vi "get_19052_AC_step_test_time.vi"(8 "error in (no error)":errorcluster, 10 "Step":u16=1 min=1 max=99 step=1, 11 "VISA resource in":refnum<visa-resource-name>) -> (0 "error out":errorcluster, 2 "AC total time":string, 3 "VISA resource out":refnum<visa-resource-name>)   [LabVIEW 2015]
doc: "This VI retrieves the test TIME of the selected step and mode."
uses:
  Type Definitions/get_19052_AC_step_time_states.ctl
  Type Definitions/ac_dc_ir_control.ctl
panel:
  # "Get 19052 AC test time"
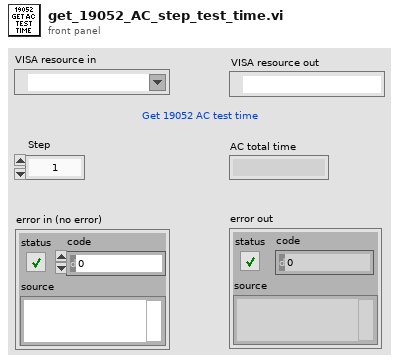
[diagram p1: front panel]
types:
  T1 = typedef "get_19052_AC_step_time_states.ctl" = enum16{"Initilize", "get RAMP time", "get TIME", "get FALL time", "calc TOTAL time", "Error", "Shutdown"}
  T2 = cluster{"ramp time":dbl, "time":dbl, "fall time":dbl, "total time":string}
  T3 = typedef "ac_dc_ir_control.ctl" = enum16{"AC", "DC", "IR"}
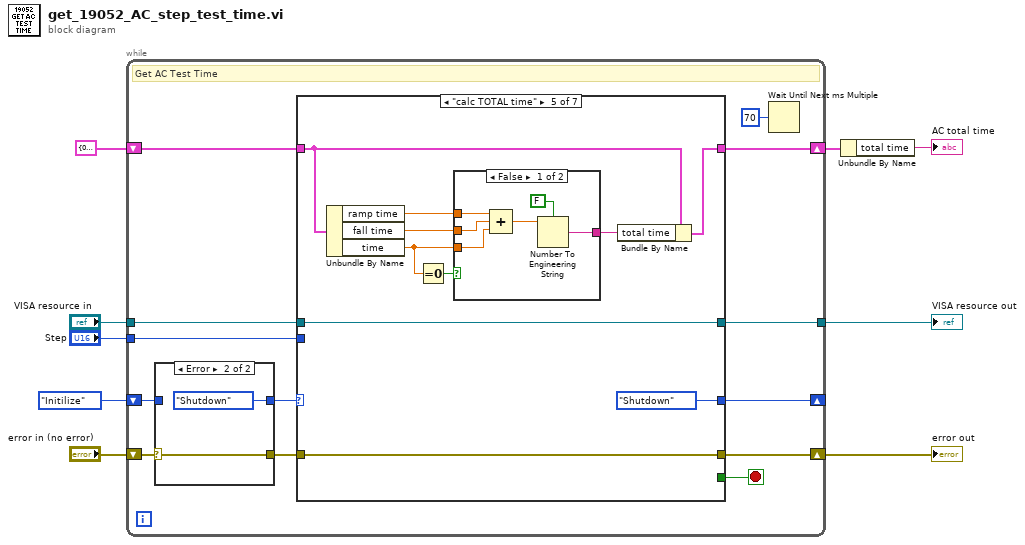
[diagram p0: block diagram]
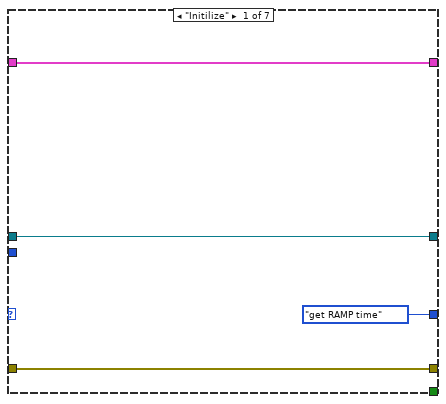
[diagram p3: hidden frame]
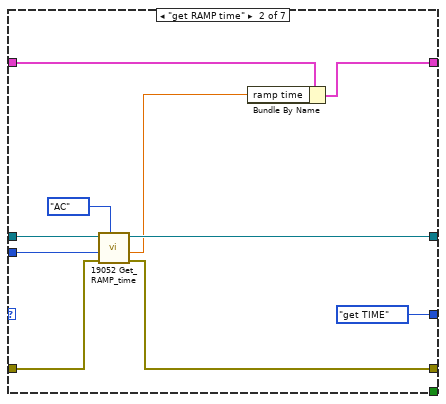
[diagram p4: hidden frame]
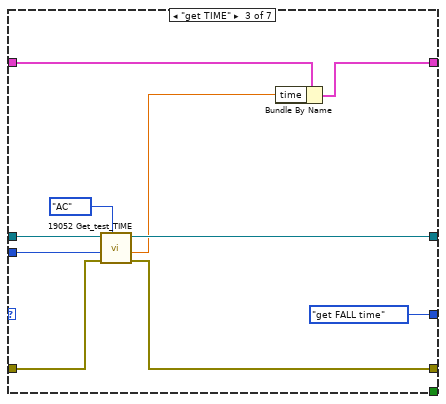
[diagram p5: hidden frame]
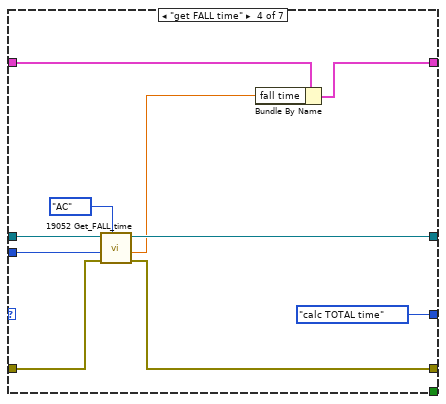
[diagram p6: hidden frame]
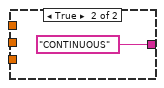
[diagram p7: hidden frame]
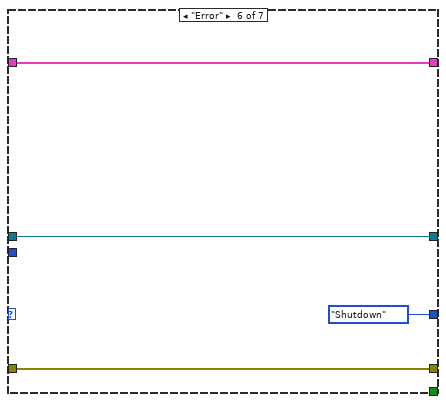
[diagram p8: hidden frame]
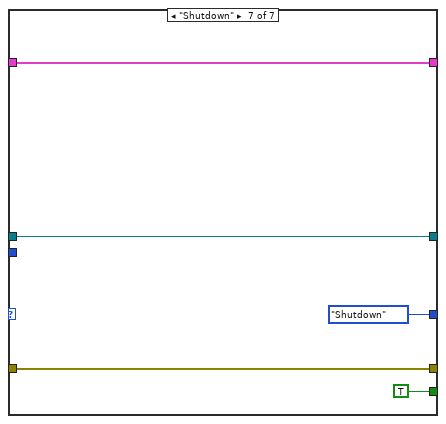
[diagram p9: hidden frame]
diagram:
  n1 = while {
    shift-right: [w22] -> _
    shift-left: get_19052_AC_step_time_states."Initilize" ("States") -> [w13]
    tunnel: "VISA resource in" -> [w21]
    tunnel: [w20] -> w6
    shift-right: [w19] -> w8
    shift-left: "error in (no error)" -> [w16]
    shift-right: [w17] -> w2
    shift-left: T2 {"ramp time"=0.0, "time"=0.0, "fall time"=0.0, "total time"=""} -> [w18]
    tunnel: "Step" -> [w12]
    stop <- w11 stop-if-true
    # "Get AC Test Time"
    n2 = case shown="Error" w16 {
      selector: w16 -> [w24 w26]
      tunnel: [w24 w26] -> w15
      tunnel: [w23 get_19052_AC_step_time_states."Shutdown" ("States")] -> w14
      tunnel: w13 -> [w23 _]
      frame No Error {
      }
      frame Error {
      }
    }
    n3 = case shown="\"calc TOTAL time\"" w14 {
      tunnel: [get_19052_AC_step_time_states."get RAMP time" ("States") get_19052_AC_step_time_states."get TIME" ("States") get_19052_AC_step_time_states."get FALL time" ("States") get_19052_AC_step_time_states."calc TOTAL time" ("States") get_19052_AC_step_time_states."Shutdown" ("States") get_19052_AC_step_time_states."Shutdown" ("States") get_19052_AC_step_time_states."Shutdown" ("States")] -> w22
      tunnel: w21 -> [w30 w39 w48 w58 w70 w81 w86]
      tunnel: [w30 w38 w46 w56 w70 w81 w86] -> w20
      tunnel: w15 -> [w29 w37 w47 w57 w69 w80 w85]
      tunnel: [w29 w36 w45 w55 w69 w80 w85] -> w19
      tunnel: w18 -> [w28 w40 w50 w60 w66 w79 w84]
      tunnel: [w28 w34 w49 w59 w67 w79 w84] -> w17
      tunnel: w12 -> [_ w35 w44 w54 _ _ _]
      tunnel: [_ _ _ _ _ _ TRUE] -> w11
      frame "Initilize" {
      }
      frame "get RAMP time" {
        n4 = call "19052 Get_RAMP_time.vi"("Mode"=ac_dc_ir_control."AC", "error in (no error)"=w37, "Step"=w35, "VISA resource in"=w39) -> ("error out"=w36:errorcluster, "RAMP time"=w33:dbl, "VISA resource out"=w38:refnum<visa-resource-name>)  [unwired: 5 in]
        n5 = Bundle By Name(cluster=w40, "ramp time"=w33) -> (w34:T2)
      }
      frame "get TIME" {
        n6 = call "19052 Get_test_TIME.vi"("Mode"=ac_dc_ir_control."AC", "error in (no error)"=w47, "Step"=w44, "VISA resource in"=w48) -> ("error out"=w45:errorcluster, "Test TIME"=w43:dbl, "VISA resource out"=w46:refnum<visa-resource-name>)  [unwired: 5 in]
        n7 = Bundle By Name(cluster=w50, "time"=w43) -> (w49:T2)
      }
      frame "get FALL time" {
        n8 = call "19052 Get_FALL_time.vi"("Mode"=ac_dc_ir_control."AC", "error in (no error)"=w57, "Step"=w54, "VISA resource in"=w58) -> ("error out"=w55:errorcluster, "FALL time"=w53:dbl, "VISA resource out"=w56:refnum<visa-resource-name>)  [unwired: 5 in]
        n9 = Bundle By Name(cluster=w60, "fall time"=w53) -> (w59:T2)
      }
      frame "calc TOTAL time" {
        n10 = Unbundle By Name(w66) -> ("ramp time"=w62:dbl, "fall time"=w63:dbl, "time"=w64:dbl)
        n11 = Equal To 0?(x=w64) -> (x = 0?=w65:bool)
        n12 = case shown="False" w65 {
          tunnel: w64 -> [w74 _]
          tunnel: w63 -> [w73 _]
          tunnel: w62 -> [w72 _]
          tunnel: [w71 "CONTINUOUS"] -> w61
          frame False {
            n13 = Compound Arithmetic op=ADD(w72, w73, w74) -> (w76:dbl)
            n14 = Number To Engineering String(1:FALSE ("use system decimal point (T)"), 4:w76) -> (0:w71:string)  [unwired: 2 in]
          }
          frame True {
          }
        }
        n15 = Bundle By Name(cluster=w66, "total time"=w61) -> (w67:T2)
      }
      frame "Error" {
      }
      frame "Shutdown" {
      }
    }
    n16 = Wait Until Next ms Multiple(millisecond multiple=u32 70) -> ()  [unwired: 1 out]
  }
  "error out" <- w8
  "VISA resource out" <- w6
  n17 = Unbundle By Name(w2) -> ("total time"=→"AC total time":string)
